vi "MicroPulse - decode amp-reporting mode.vi"(1 "Byte0":u8, 2 "Byte 1":u8, 3 "Byte 2":u8, 4 "Byte 3":u8) -> (0 "script":string)   [LabVIEW 2026, in "MicroPulse_Driver.lvlib"]
uses:
  MicroPulse_Driver.lvlib
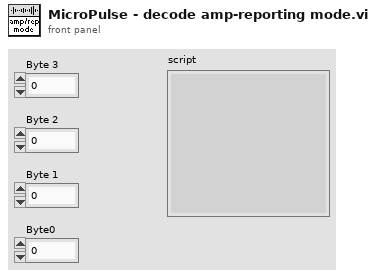
[diagram p1: front panel]
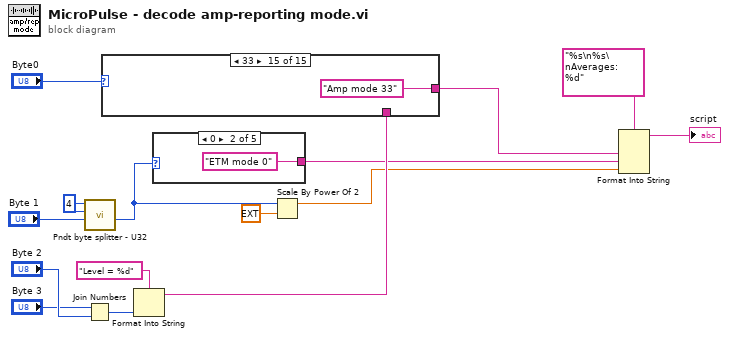
[diagram p0: block diagram]
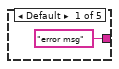
[diagram p2: hidden frame]
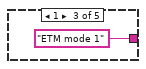
[diagram p3: hidden frame]
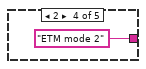
[diagram p4: hidden frame]
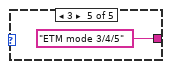
[diagram p5: hidden frame]
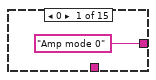
[diagram p6: hidden frame]
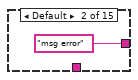
[diagram p7: hidden frame]
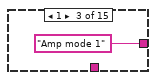
[diagram p8: hidden frame]
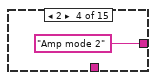
[diagram p9: hidden frame]
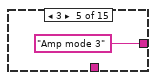
[diagram p10: hidden frame]
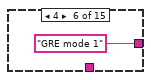
[diagram p11: hidden frame]
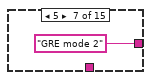
[diagram p12: hidden frame]
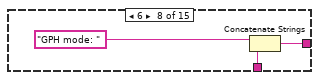
[diagram p13: hidden frame]
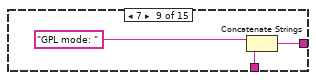
[diagram p14: hidden frame]
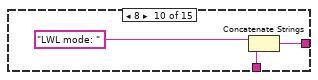
[diagram p15: hidden frame]
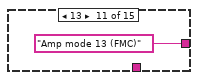
[diagram p16: hidden frame]
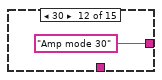
[diagram p17: hidden frame]
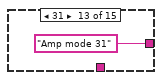
[diagram p18: hidden frame]
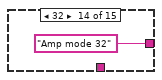
[diagram p19: hidden frame]
diagram:
  w6 = i16 4 ("shift right")
  n1 = call "Pndt byte splitter - U32.vi"("byte U32"="Byte 1", "mask size"=w6, "shift right"=w6) -> ("lo"=w2:u32)  [unwired: 7 in, 1 out]
  n2 = Join Numbers(hi="Byte 3", lo="Byte 2") -> ((hi.lo)=w9:u16)
  n3 = Format Into String(format string="Level = %d", w9) -> (resulting string=w7:string)  [unwired: 2 in, 1 out]
  n4 = case shown="33" "Byte0" {
    tunnel: ["Amp mode 0" "msg error" "Amp mode 1" "Amp mode 2" "Amp mode 3" "GRE mode 1" "GRE mode 2" w24 w27 w30 "Amp mode 13 (FMC)" "Amp mode 30" "Amp mode 31" "Amp mode 32" "Amp mode 33"] -> w12
    tunnel: w7 -> [_ _ _ _ _ _ _ w23 w26 w29 _ _ _ _ _]
    frame 0 {
    }
    frame Default {
    }
    frame 1 {
    }
    frame 2 {
    }
    frame 3 {
    }
    frame 4 {
    }
    frame 5 {
    }
    frame 6 {
      n5 = Concatenate Strings("GPH mode: ", w23) -> (w24:string)
    }
    frame 7 {
      n6 = Concatenate Strings("GPL mode: ", w26) -> (w27:string)
    }
    frame 8 {
      n7 = Concatenate Strings("LWL mode: ", w29) -> (w30:string)
    }
    frame 13 {
    }
    frame 30 {
    }
    frame 31 {
    }
    frame 32 {
    }
    frame 33 {
    }
  }
  n8 = case shown="0" w2 {
    tunnel: ["error msg" "ETM mode 0" "ETM mode 1" "ETM mode 2" "ETM mode 3/4/5"] -> w4
    frame Default {
    }
    frame 0 {
    }
    frame 1 {
    }
    frame 2 {
    }
    frame 3 {
    }
  }
  n9 = Scale By Power Of 2(n=w2, x=ext 1.0) -> (x*2^n=w3:ext)
  n10 = Format Into String(format string="%s\n%s\nAverages:  %d", w12, w4, w3) -> (resulting string=→"script":string)  [unwired: 2 in, 1 out]
